vi "Create Tree & Node Values.vi"(8 "error in (no error)":errorcluster, 10 "Letters to code":string[](array[string]), 11 "Linked Nodes IN":T1[](array[typedef])) -> (0 "error out":errorcluster, 3 "Huffman codes for each letter":string[][](array[string]))   [LabVIEW 2017]
uses:
  BinaryNode.ctl
panel:
  out "Huffman codes for each node":string[][](array[string])
  out "Created Tree":string(tree)
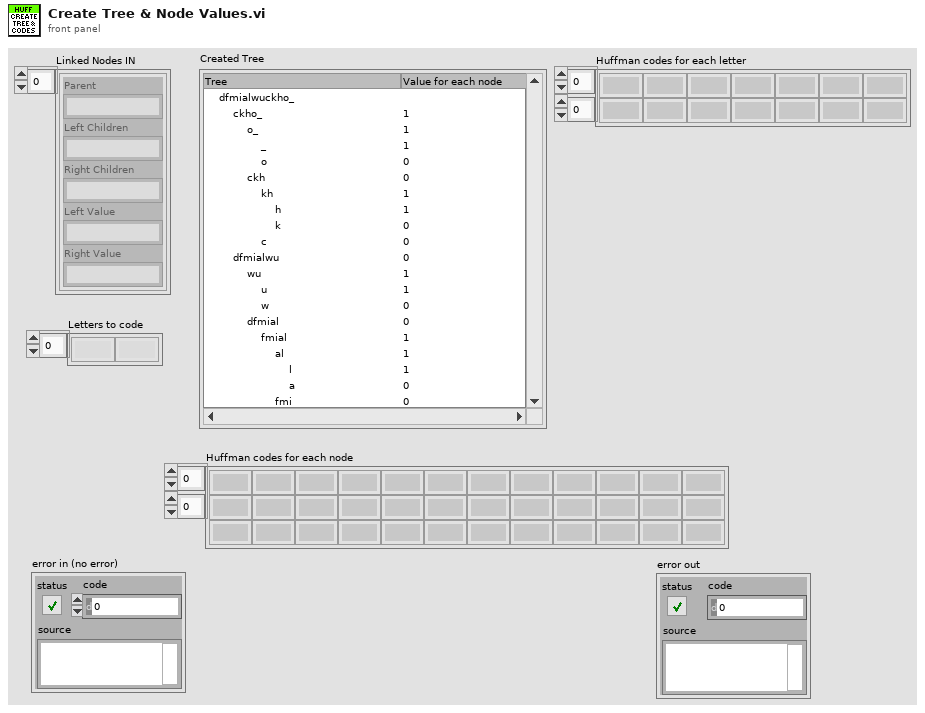
[diagram p1: front panel]
types:
  T1 = typedef "BinaryNode.ctl" = cluster{"Parent":string, "Left Children":string, "Right Children":string, "Left Value":string, "Right Value":string}
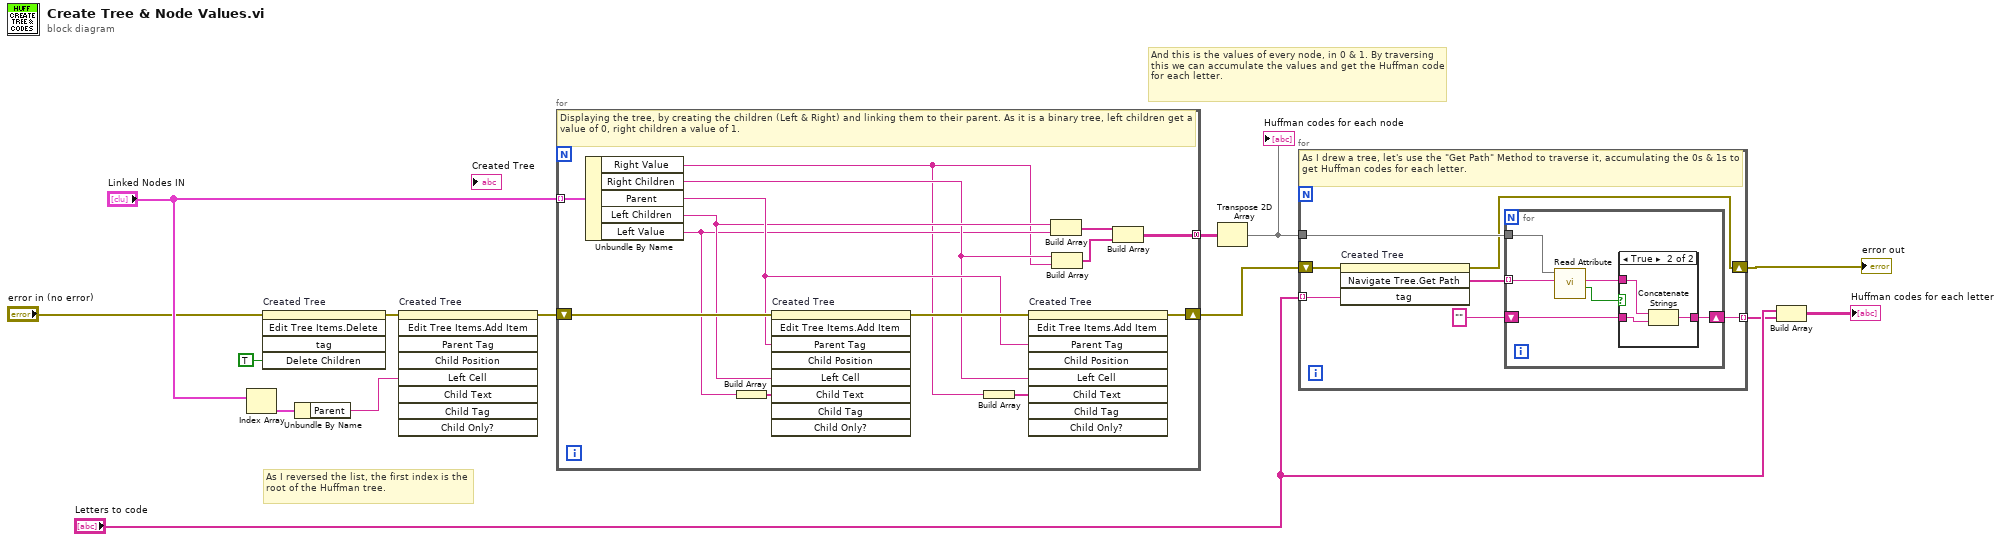
[diagram p0: block diagram]
diagram:
  # "And this is the values of every node, in 0 & 1. By traversing this we can accumulate the values and get the Huffman code for each letter."
  # "As I reversed the list, the first index is the root of the Huffman tree."
  n1 = Index Array(array="Linked Nodes IN") -> (element=w6:T1)  [unwired: 1 in]
  n2 = invoke on="Created Tree" class="Tree (strict)" method="Edit Tree Items.Delete"(error in="error in (no error)", "Delete Children"=TRUE ("Delete Children?")) -> (error out=w8:errorcluster)  [unwired: 3 in, 4 out]
  n3 = Unbundle By Name(w6) -> ("Parent"=w10:string)
  n4 = invoke on="Created Tree" class="Tree (strict)" method="Edit Tree Items.Add Item"(error in=w8, "Left Cell"=w10) -> (error out=w7:errorcluster)  [unwired: 7 in, 8 out]
  n5 = for {
    tunnel: "Linked Nodes IN" -> [w25] mode=indexing
    shift-right: [w26] -> w2
    shift-left: w7 -> [w28]
    tunnel: [w21] -> w11 mode=concatenating
    # "Displaying the tree, by creating the children (Left & Right) and linking them to their parent. As it is a binary tree, left children get a value of 0, right children a value of 1."
    n6 = Unbundle By Name(w25) -> ("Right Value"=w15:string, "Right Children"=w19:string, "Parent"=w24:string, "Left Children"=w20:string, "Left Value"=w18:string)
    n7 = Build Array(w18) -> (w17:string[])
    n8 = invoke on="Created Tree" class="Tree (strict)" method="Edit Tree Items.Add Item"(error in=w28, "Parent Tag"=w24, "Left Cell"=w20, "Child Text"=w17) -> (error out=w27:errorcluster)  [unwired: 5 in, 8 out]
    n9 = Build Array(w15) -> (w16:string[])
    n10 = invoke on="Created Tree" class="Tree (strict)" method="Edit Tree Items.Add Item"(error in=w27, "Parent Tag"=w24, "Left Cell"=w19, "Child Text"=w16) -> (error out=w26:errorcluster)  [unwired: 5 in, 8 out]
    n11 = Build Array(w20, w18) -> (w23:string[])
    n12 = Build Array(w19, w15) -> (w22:string[])
    n13 = Build Array(w23, w22) -> (w21:string[][])
  }
  n14 = Transpose 2D Array(2D array=w11) -> (transposed array=w3:string[][])
  "Huffman codes for each node" <- w3
  n15 = for {
    tunnel: [w33] -> w12 mode=indexing
    tunnel: w3 -> [w32]
    tunnel: "Letters to code" -> [w29] mode=indexing
    shift-right: [w30] -> w1
    shift-left: w2 -> [w31]
    # "As I drew a tree, let's use the \"Get Path\" Method to traverse it, accumulating the 0s & 1s to get Huffman codes for each letter."
    n16 = invoke on="Created Tree" class="Tree (strict)" method="Navigate Tree.Get Path"(error in=w31, "tag"=w29) -> (error out=w30:errorcluster, "Navigate Tree:Get Path"=w35:string[])  [unwired: 2 in, 2 out]
    n17 = for {
      tunnel: w35 -> [w38] mode=indexing
      shift-right: [w40] -> w33
      shift-left: "" -> [w41]
      tunnel: w32 -> [w39]
      n18 = call "Read Attribute.vi"("Attribute to Read"=w38, "Object Attributes IN"=w39) -> ("Found?"=w37:bool, "Attribute Value"=w36:string)  [unwired: 7 in, 1 out]
      n19 = case shown="True" w37 {
        tunnel: w41 -> [w42 w45]
        tunnel: [w42 w44] -> w40
        tunnel: w36 -> [_ w43]
        frame False {
        }
        frame True {
          n20 = Concatenate Strings(w43, w45) -> (w44:string)
        }
      }
    }
  }
  "error out" <- w1
  n21 = Build Array("Letters to code", w12) -> (→"Huffman codes for each letter":string[][])
